vi "sysconfig initialize benchmark.vi"() -> ()   [LabVIEW 2017]
uses:
  <vilib>/nisyscfg/Language.ctl
  <vilib>/nisyscfg/nisyscfg.lvlib
panel:
  out "time":dbl=21.13189935684204
  out "Session out":refnum<k21>="10.118.8.70"
  out "error out":errorcluster={"status"=TRUE, "code"=-2147220621, "source"="nisyscfg.lvlib:Initialize (Helper).vi:3930001<APPEND>\n\n<b>Complete call chain:</b>\r\n     nisyscfg.lvlib:Initialize (Helper).vi:3930001\r\n     nisyscfg.lvlib:Initialize Session.vi:1230001\r\n     sysconfig initialize benchmark.vi"}
  in  "Target (localhost)":refnum<k21>="10.118.8.70"
  in  "Force Property Refresh (T)":bool=TRUE
  in  "Language (Automatic)":T1 items=["Automatic"=0, "Chinese Simplified"=2052, "English"=1033, "French"=1036, "German"=1031, "Japanese"=1041, "Korean"=1042]
  in  "error in (no error)":errorcluster
  in  "User Name":string
  in  "Connect Timeout (4000 ms)":u32=4000
  in  "Password":string
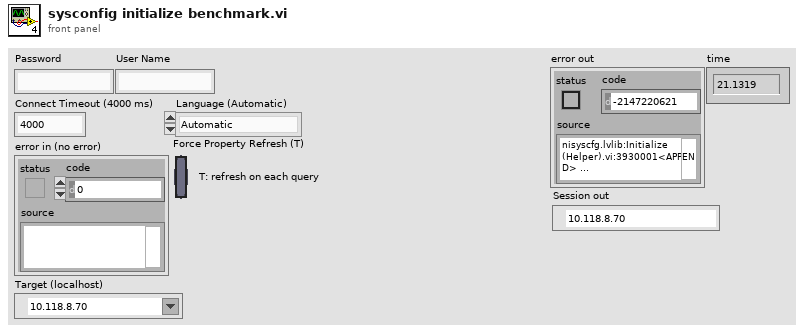
[diagram p1: front panel]
types:
  T1 = typedef "nisyscfg.lvlib/Language.ctl" = i32
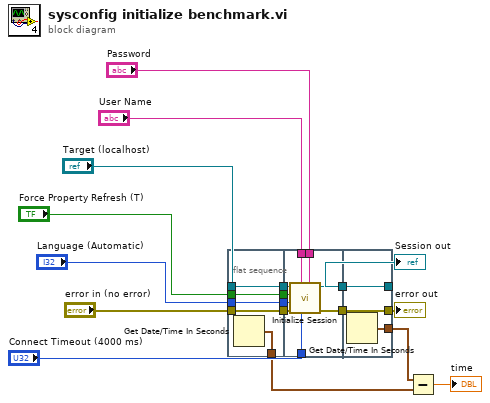
[diagram p0: block diagram]
diagram:
  n1 = flat-sequence {
    tunnel: "Target (localhost)" -> [w20]
    tunnel: "Force Property Refresh (T)" -> [w21]
    tunnel: "Language (Automatic)" -> [w22]
    tunnel: "error in (no error)" -> [w23]
    tunnel: [w23] -> w9
    tunnel: [w22] -> w8
    tunnel: [w21] -> w7
    tunnel: [w20] -> w6
    tunnel: [w19] -> w2
    tunnel: "Password" -> [w32]
    tunnel: "Connect Timeout (4000 ms)" -> [w31]
    tunnel: "User Name" -> [w30]
    tunnel: w9 -> [w29]
    tunnel: w8 -> [w28]
    tunnel: w7 -> [w27]
    tunnel: w6 -> [w26]
    tunnel: [w25] -> w5
    tunnel: [w24] -> w4
    tunnel: [w34] -> w10
    tunnel: [w35] -> w11
    tunnel: w5 -> [w35]
    tunnel: w4 -> [w34]
    tunnel: [w33] -> w3
    frame #0 {
      n2 = Get Date/Time In Seconds() -> (seconds since 1Jan1904=w19:timestamp)
    }
    frame #1 {
      n3 = call <vilib>:"Initialize Session.vi"("Password"=w32, "Connect Timeout (4000 ms)"=w31, "User Name"=w30, "error in (no error)"=w29, "Language (Automatic)"=w28, "Force Property Refresh (T)"=w27, "Target (localhost)"=w26) -> ("error out"=w25:errorcluster, "Session out"=w24:refnum<k21>)  [unwired: 3 in]
    }
    frame #2 {
      n4 = Get Date/Time In Seconds() -> (seconds since 1Jan1904=w33:timestamp)
    }
  }
  n5 = Subtract(x=w3, y=w2) -> (x-y=→"time":dbl)
  "error out" <- w11
  "Session out" <- w10
